vi "UMDLoopTelem.vi"   [LabVIEW 2017]
types:
  T1 = cluster{"X dtheta":sgl, "Y dtheta":sgl, "Z dtheta":sgl, "X accel":sgl, "Y accel":sgl, "Z accel":sgl, "Velocity":sgl, "IMU Fault":bool, "Time Since Last Tape":sgl, "Position":sgl}
  T2 = cluster{"Primary Battery 1 Voltage":sgl, "Primary Battery 2 Voltage":sgl, "Reserve Battery Voltage":sgl, "Primary Battery 1 Current":sgl, "Primary Battery 2 Current":sgl, "Reserve Battery Current":sgl, "Primary Battery 1 Temperature":sgl, "Primary Battery 2 Temperature":sgl, "Reserve Battery Temperature":sgl, "Primary Battery 1 Low":bool, "Primary Battery 2 Low":bool, "Reserve Battery Low":bool, "Primary Battery 1 Critical":bool, "Primary Battery 2 Critical":bool, "Reserve Battery Critical":bool, "Primary Battery 1 Hot":bool, "Primary Battery 2 Hot":bool, "Reserve Battery Hot":bool, "Frame Temperature":sgl, "Frame Hot":bool, "Ambient Pressure":sgl, "Tank Pressure":sgl, "Downstream Pressure":sgl, "Tank Pressue Low":bool, "Downstream Pressure Low":bool, "Tank Pressure Fault":bool, "Downstream Pressure Fault":bool, "IR 1 RAW":sgl, "IR 2 RAW":sgl, "IR Fault":bool, "Pusher Connected":bool, "Left Tape Count":u32, "Right Tape Count":u32, "Left Velocity":sgl, "Right Velocity":sgl, "Left LS Fault":bool, "Right LS Fault":bool, "Levitation Height":sgl, "Levitating?":bool, "PCS 1 Position":sgl, "PCS 2 Position":sgl, "PCS 3 Position":sgl, "PCS 4 Position":sgl, "FL Count":u8, "FR Count":u8, " BL Count":u8, "BR Count":u8}
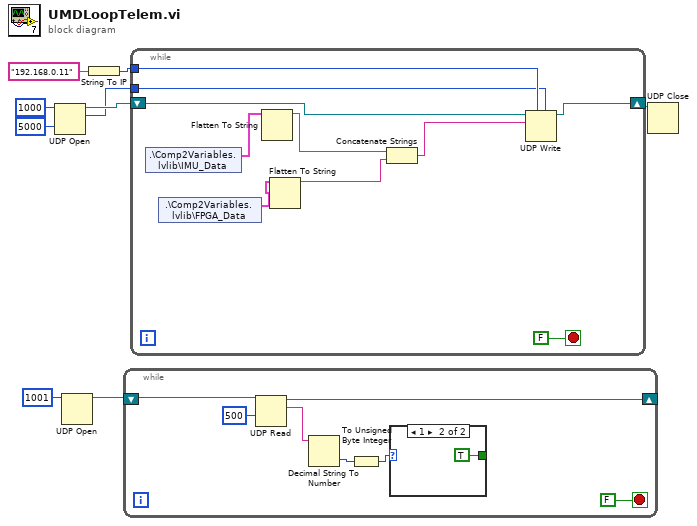
[diagram p0: block diagram]
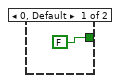
[diagram p2: hidden frame]
diagram:
  n1 = UDP Open(9:5000 ("timeout ms (25000)"), 11:u16 1000 ("port")) -> (port=w9:refnum<k16>, 2:w5:u16)  [unwired: 3 in, 1 out]
  n2 = UDP Open(11:u16 1001 ("port")) -> (port=w2:refnum<k16>)  [unwired: 4 in, 2 out]
  n3 = String To IP(1:"192.168.0.11" ("name")) -> (0:w8:u32)
  n4 = while {
    shift-right: [w10] -> _
    shift-left: w2 -> [w11]
    stop <- FALSE stop-if-true
    n5 = UDP Read(connection ID=w11, timeout ms (25000)=500) -> (data out=w14:string, 3:w10:refnum<k16>)  [unwired: 2 in, 3 out]
    n6 = Decimal String To Number(string=w14) -> (number=w15:i32)  [unwired: 2 in, 1 out]
    n7 = To Unsigned Byte Integer(number=w15) -> (unsigned 8bit integer=w13:u8)
    n8 = case shown="1" w13 {
      tunnel: [FALSE TRUE] -> _
      frame 0, Default {
      }
      frame 1 {
      }
    }
  }
  n9 = while {
    tunnel: w8 -> [w25]
    tunnel: w5 -> [w24]
    shift-right: [w26] -> w3
    shift-left: w9 -> [w27]
    stop <- FALSE stop-if-true
    n10 = shared-variable ".\\Comp2Variables.lvlib\\IMU_Data"() -> (w23:T1)  [unwired: 1 in, 1 out]
    n11 = shared-variable ".\\Comp2Variables.lvlib\\FPGA_Data"() -> (w22:T2)  [unwired: 1 in, 1 out]
    n12 = Flatten To String(anything=w23) -> (data string=w21:string)  [unwired: 3 in, 2 out]
    n13 = Flatten To String(anything=w22) -> (data string=w20:string)  [unwired: 3 in, 2 out]
    n14 = Concatenate Strings(w21, w20) -> (w19:string)
    n15 = UDP Write(address=w25, port or service name=w24, connection ID=w27, data in=w19) -> (3:w26:refnum<k16>)  [unwired: 2 in, 1 out]
  }
  n16 = UDP Close(connection ID=w3) -> ()  [unwired: 1 in, 2 out]
